vi "ControllerMain.vi"(8 "Error In":errorcluster, 11 "Control Mode":T4(ring)) -> (0 "Error Out":errorcluster, 3 "Robot Inputs":T3, 4 "Joystick1DevRef":T1={"Device"=enum."USB 1"}, 5 "Stick0 Buttons":bool[](array[boolean]), 6 "Joystick0DevRef":T1={"Device"=enum."USB 1"}, 7 "Stick0 Axes":dbl[](array[numeric]))   [LabVIEW 2017]
uses:
  TeleopCommands.ctl
  <vilib>/Rock Robotics/WPI/Joystick/WPI_JoystickDevRef.ctl
  <vilib>/Rock Robotics/WPI/Joystick/WPI_JoystickDeviceEnum.ctl
  <vilib>/Rock Robotics/WPI/Utilities/WPI_GetSetVariantRefNum.vi
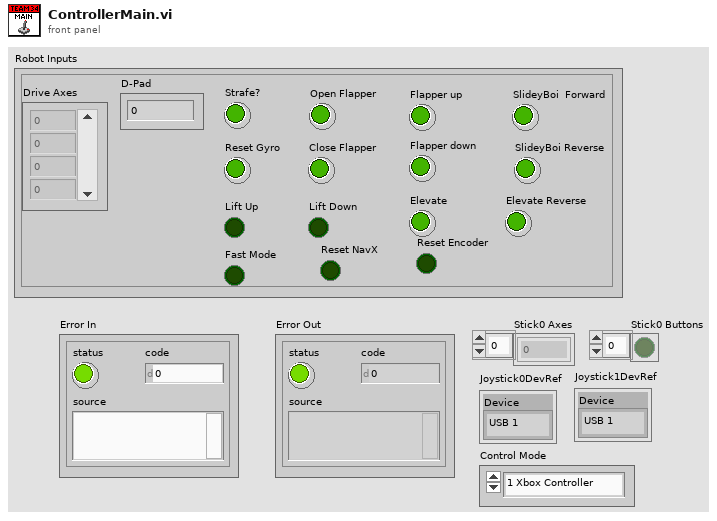
[diagram p1: front panel]
types:
  T1 = typedef "WPI_JoystickDevRef.ctl" = cluster{"Device":T2}
  T2 = typedef "WPI_JoystickDeviceEnum.ctl" = enum16{"USB 0", "USB 1", "USB 2", "USB 3", "USB 4", "USB 5"}
  T3 = typedef "TeleopCommands.ctl" = cluster{"Drive Axes":dbl[], "Reset Gyro":bool, "Strafe?":bool, "Open Flapper":bool, "Close Flapper":bool, "Flapper up":bool, "Flapper down":bool, "D-Pad":i64, "SlideyBoi  Forward":bool, "SlideyBoi Reverse":bool, "Lift Up":bool, "Lift Down":bool, "Elevate":bool, "Elevate Reverse":bool, "Fast Mode":bool, "Reset NavX":bool, "Reset Encoder":bool}
  T4 = enum16{"1 Xbox Controller", "2 Xbox Controllers"}
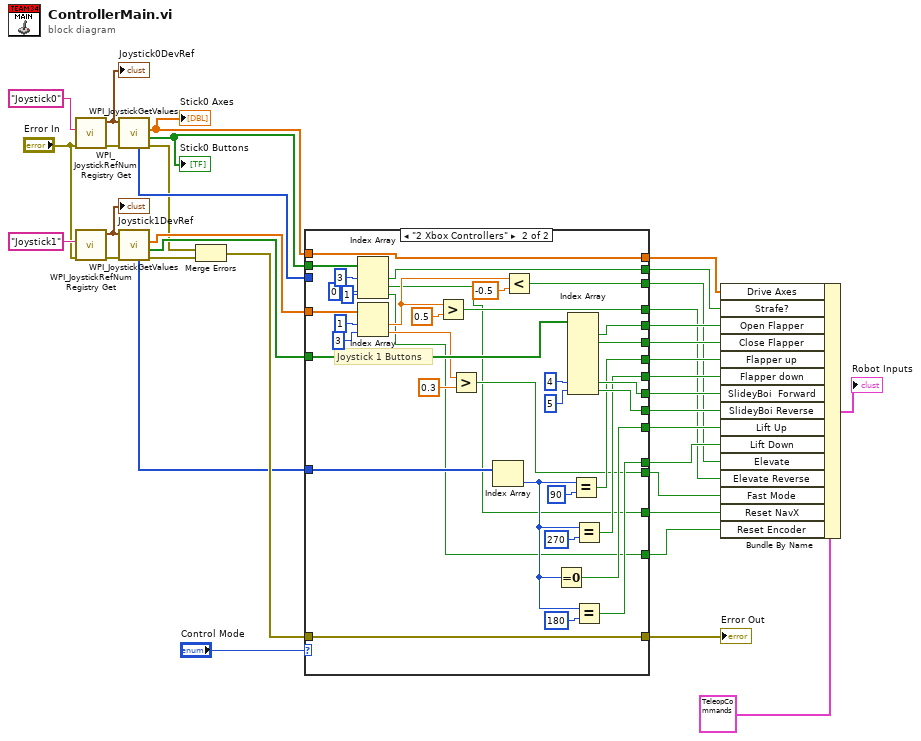
[diagram p0: block diagram]
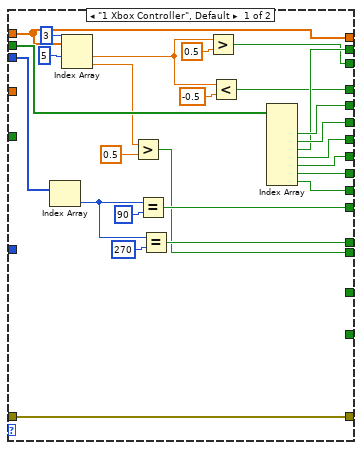
[diagram p2: hidden frame]
diagram:
  n1 = call <vilib>:"WPI_JoystickRefNum Registry Get.vi"("error in (no error)"="Error In", "refnum name"="Joystick0") -> ("error out"=w30:errorcluster, "JoystickDevRef"=w35:T1)  [unwired: 8 out]
  "Joystick0DevRef" <- w35
  n2 = call <vilib>:"WPI_JoystickRefNum Registry Get.vi"("error in (no error)"="Error In", "refnum name"="Joystick1") -> ("error out"=w31:errorcluster, "JoystickDevRef"=w32:T1)  [unwired: 8 out]
  "Joystick1DevRef" <- w32
  n3 = call <vilib>:"WPI_JoystickGetValues.vi"("error in (no error)"=w30, "JoystickDevRef"=w35) -> ("error out"=w21:errorcluster, "Buttons"=w27:bool[], "Axes"=w28:dbl[], "POVs"=w23:i16[])  [unwired: 5 in, 1 out]
  "Stick0 Axes" <- w28
  "Stick0 Buttons" <- w27
  n4 = call <vilib>:"WPI_JoystickGetValues.vi"("error in (no error)"=w31, "JoystickDevRef"=w32) -> ("error out"=w20:errorcluster, "Buttons"=w26:bool[], "Axes"=w25:dbl[], "POVs"=w17:i16[])  [unwired: 5 in, 1 out]
  n5 = Merge Errors(w21, w20) -> (w19:errorcluster)
  n6 = case shown="\"2 Xbox Controllers\"" "Control Mode" {
    tunnel: w28 -> [w46 w97]
    tunnel: w27 -> [w60 w90]
    tunnel: w26 -> [_ w95]
    tunnel: w25 -> [_ w80]
    tunnel: [w46 w97] -> w24
    tunnel: w23 -> [w52 _]
    tunnel: [w61 w96] -> w18
    tunnel: w19 -> [w61 w96]
    tunnel: w17 -> [_ w94]
    tunnel: [w57 w89] -> w14
    tunnel: [w59 w88] -> w13
    tunnel: [w58 w87] -> w12
    tunnel: [w56 w71] -> w11
    tunnel: [w55 w70] -> w10
    tunnel: [w54 w93] -> w9
    tunnel: [w53 w92] -> w8
    tunnel: [w51 w73] -> w7
    tunnel: [w50 w72] -> w6
    tunnel: [w43 w74] -> w5
    tunnel: [w40 w77] -> w4
    tunnel: [w36 w66] -> w3
    tunnel: [_ w64] -> w2
    tunnel: [_ w62] -> w1
    frame "1 Xbox Controller", Default {
      n7 = Index Array(array=w52) -> (element=w49:i16)  [unwired: 1 in]
      n8 = Index Array(array=w46, index #1=5 ("index"), index #2=3 ("index")) -> (element #1=w42:dbl, element #2=w38:dbl)
      n9 = Greater?(x=w38, y=0.5) -> (0:w36:bool)
      n10 = Equal?(x=w49, y=i16 90) -> (x = y?=w51:bool)
      n11 = Equal?(x=w49, y=i16 270) -> (x = y?=w50:bool)
      n12 = Greater?(x=w42, y=0.5) -> (0:w43:bool)
      n13 = Less?(x=w42, y=-0.5) -> (x < y?=w40:bool)
      n14 = Index Array(array=w60) -> (element #2=w59:bool, element #3=w58:bool, element #4=w57:bool, element #5=w56:bool, element #6=w55:bool, element #7=w54:bool, element #8=w53:bool)  [unwired: 8 in, 1 out]
    }
    frame "2 Xbox Controllers" {
      # "Joystick 1 Buttons"
      n15 = Index Array(array=w90, index #1=3 ("index"), index #2=0 ("index"), index #3=1 ("index")) -> (element #1=w89:bool, element #2=w64:bool, element #3=w62:bool)
      n16 = Index Array(array=w80, index #1=1 ("index"), index #2=3 ("index")) -> (element #1=w76:dbl, element #2=w68:dbl)
      n17 = Greater?(x=w76, y=0.5) -> (0:w77:bool)
      n18 = Greater?(x=w68, y=0.3) -> (0:w66:bool)
      n19 = Index Array(array=w94) -> (element=w82:i16)  [unwired: 1 in]
      n20 = Less?(x=w76, y=-0.5) -> (x < y?=w74:bool)
      n21 = Equal To 0?(x=w82) -> (x = 0?=w73:bool)
      n22 = Index Array(array=w95, index #7=4 ("index"), index #8=5 ("index")) -> (element #1=w88:bool, element #2=w87:bool, element #7=w93:bool, element #8=w92:bool)  [unwired: 6 in, 4 out]
      n23 = Equal?(x=w82, y=i16 90) -> (x = y?=w71:bool)
      n24 = Equal?(x=w82, y=i16 270) -> (x = y?=w70:bool)
      n25 = Equal?(x=w82, y=i16 180) -> (x = y?=w72:bool)
    }
  }
  "Error Out" <- w18
  n26 = Bundle By Name(cluster=T3 {"Drive Axes"=[], "Reset Gyro"=FALSE, "Strafe?"=FALSE, "Open Flapper"=FALSE, "Close Flapper"=FALSE, "Flapper up"=FALSE, "Flapper down"=FALSE, "D-Pad"=0, "SlideyBoi  Forward"=FALSE, "SlideyBoi Reverse"=FALSE, "Lift Up"=FALSE, "Lift Down"=FALSE, "Elevate"=FALSE, "Elevate Reverse"=FALSE, "Fast Mode"=FALSE, "Reset NavX"=FALSE, "Reset Encoder"=FALSE} ("Robot Inputs"), "Drive Axes"=w24, "Strafe?"=w14, "Open Flapper"=w13, "Close Flapper"=w12, "Flapper up"=w11, "Flapper down"=w10, "SlideyBoi  Forward"=w9, "SlideyBoi Reverse"=w8, "Lift Up"=w7, "Lift Down"=w6, "Elevate"=w5, "Elevate Reverse"=w4, "Fast Mode"=w3, "Reset NavX"=w2, "Reset Encoder"=w1) -> (→"Robot Inputs":T3)
